vi "Demo.vi"() -> ()   [LabVIEW 2016, in "Photon Counter.lvlib" / "C8855-01.lvlib"]
uses:
  C8855-01.lvlib
  States.ctl
  Data.ctl
panel:
  out "ID":string
  in  "Counts":i32 format="%d cps"
  out "History":dbl(graph)
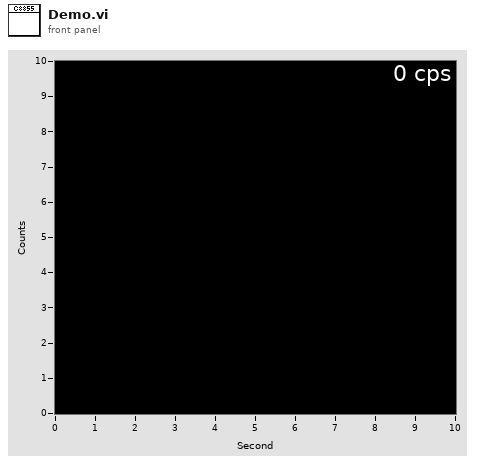
[diagram p1: front panel]
types:
  T1 = typedef "Data.ctl" = cluster{"Handle":u32}
  T2 = typedef "Photon Counter.lvlib/C8855-01.lvlib/States.ctl" = enum16{"Init", "Open", "Setup", "Idle", "Close", "Clear", "Exit"}
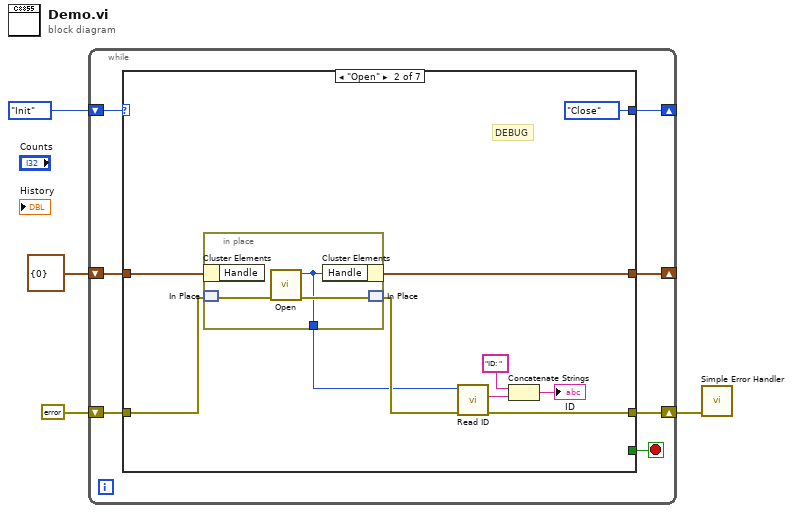
[diagram p0: block diagram]
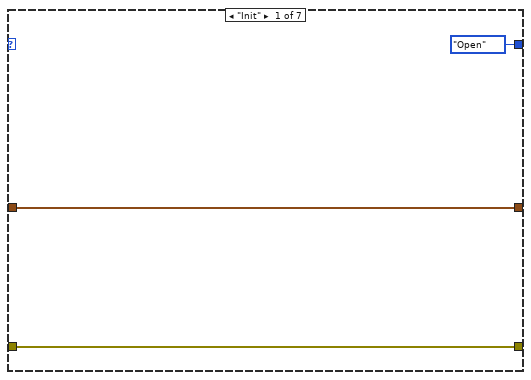
[diagram p2: hidden frame]
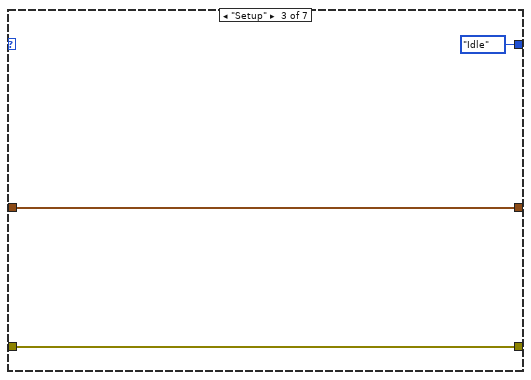
[diagram p3: hidden frame]
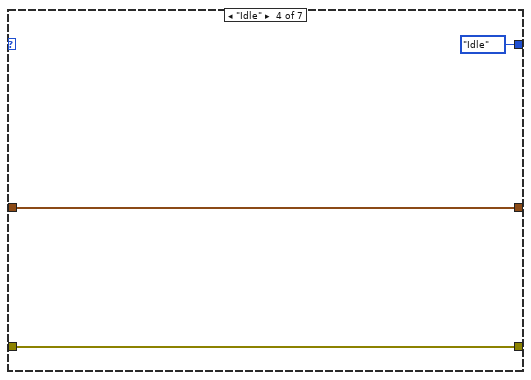
[diagram p4: hidden frame]
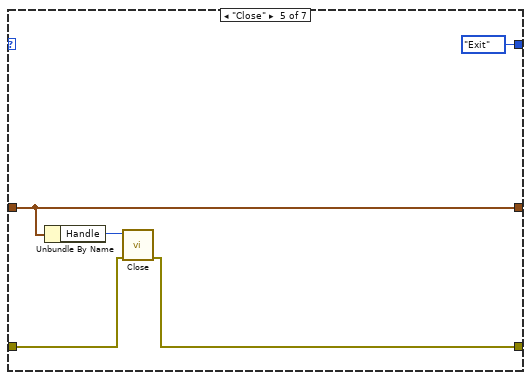
[diagram p5: hidden frame]
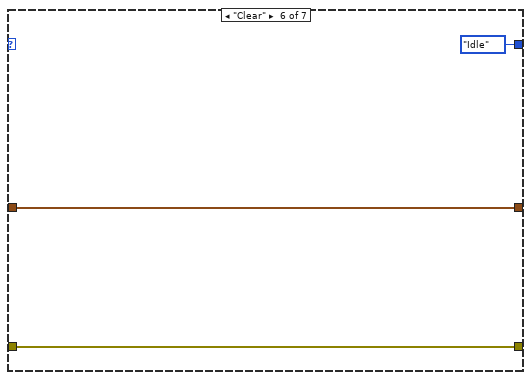
[diagram p6: hidden frame]
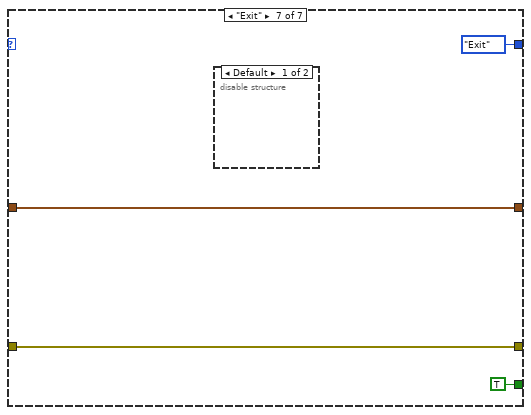
[diagram p7: hidden frame]
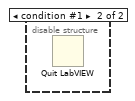
[diagram p8: hidden frame]
diagram:
  n1 = while {
    shift-right: [w9] -> _
    shift-left: States."Init" -> [w10]
    shift-right: [w5] -> w1
    shift-left: errorcluster {"status"=FALSE, "code"=0, "source"=""} ("error in (no error)") -> [w8]
    shift-right: [w6] -> _
    shift-left: T1 {"Handle"=0} -> [w7]
    stop <- w11 stop-if-true
    n2 = case shown="\"Open\"" w10 {
      tunnel: [_ _ _ _ _ _ TRUE] -> w11
      tunnel: [States."Open" States."Close" States."Idle" States."Idle" States."Exit" States."Idle" States."Exit"] -> w9
      tunnel: w8 -> [w13 w21 w29 w32 w35 w39 w44]
      tunnel: w7 -> [w12 w23 w28 w31 w37 w40 w42]
      tunnel: [w12 w22 w28 w31 w37 w40 w42] -> w6
      tunnel: [w13 w19 w29 w32 w34 w39 w44] -> w5
      frame "Init" {
      }
      frame "Open" {
        # "DEBUG"
        n3 = in-place {
          in-place-border: [w25] -> w18
          n4 = in-place-cluster #1(w23) -> ()  [unwired: 1 out]
          n5 = in-place-match #2(w21) -> (w26:errorcluster)
          n6 = call "Open.vi"("error in (no error)"=w26) -> ("error out"=w27:errorcluster, "Handle"=w25:u32)  [unwired: 9 in]
          n7 = in-place-cluster #1("Handle"=w25) -> (w22:T1)
          n8 = in-place-match #2(w27) -> (w20:errorcluster)
        }
        n9 = call "Read ID.vi"("error in (no error)"=w20, "Handle"=w18) -> ("error out"=w19:errorcluster, "Data"=w17:string)  [unwired: 7 in, 1 out]
        n10 = Concatenate Strings("ID: " ("string"), w17) -> (→"ID":string)
      }
      frame "Setup" {
      }
      frame "Idle" {
      }
      frame "Close" {
        n11 = Unbundle By Name(w37) -> ("Handle"=w36:u32)
        n12 = call "Close.vi"("error in (no error)"=w35, "Handle"=w36) -> ("error out"=w34:errorcluster)  [unwired: 8 in, 1 out]
      }
      frame "Clear" {
      }
      frame "Exit" {
        n13 = disable-structure shown="Default" {
          frame condition #0 (active) {
          }
          frame condition #1 {
            n14 = Quit LabVIEW() -> ()  [unwired: 1 in]
          }
        }
      }
    }
  }
  n15 = call <vilib>:"Simple Error Handler.vi"("error in (no error)"=w1) -> ()  [unwired: 4 in, 5 out]
